vi "Creat file.vi"(10 "Numeric":i32, 11 "File Path":string) -> (3 "Path":path)   [LabVIEW 2011]
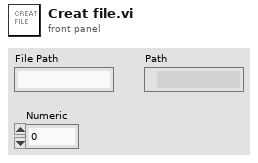
[diagram p1: front panel]
types:
  T1 = enum16{"open", "replace", "create", "open or create", "replace or create", "replace or create with confirmation"}
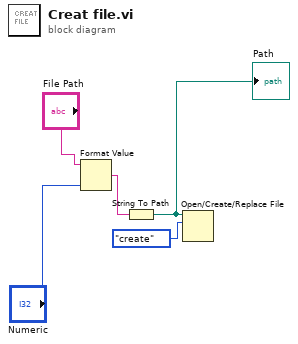
[diagram p0: block diagram]
diagram:
  n1 = Format Value(string ("")="File Path", value (0)="Numeric") -> (output string=w2:string)  [unwired: 1 in]
  n2 = String To Path(string=w2) -> (path=w5:path)
  "Path" <- w5
  n3 = Open/Create/Replace File(file path (use dialog)=w5, operation (0:open)=T1."create") -> ()  [unwired: 4 in, 3 out]
